vi "Мультиплексор(2 5-разрядных операнда).vi"(1 "c":bool, 2 "Inp1":T2, 3 "Inp0":T2) -> (0 "r":T1)   [LabVIEW 2013]
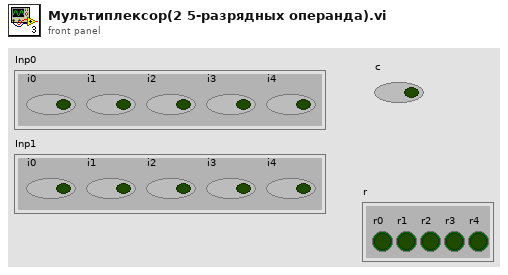
[diagram p1: front panel]
types:
  T1 = cluster{"r0":bool, "r1":bool, "r2":bool, "r3":bool, "r4":bool}
  T2 = cluster{"i0":bool, "i1":bool, "i2":bool, "i3":bool, "i4":bool}
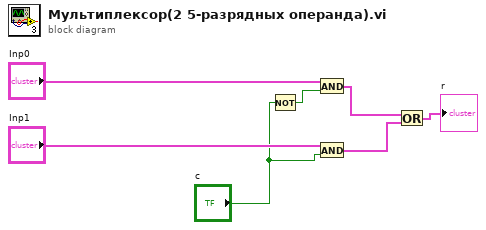
[diagram p0: block diagram]
diagram:
  n1 = Not(x="c") -> (.not. x?=w2:bool)
  n2 = And(x="Inp0", y=w2) -> (x .and. y?=w5:T2)
  n3 = And(x="Inp1", y="c") -> (x .and. y?=w4:T2)
  n4 = Or(x=w5, y=w4) -> (x .or. y?=→"r":T2)
